vi "Set Injected Value.vi"(8 "error in (no error)":errorcluster, 10 "Value":T1, 11 "Fault-Injection_Boolean in":refnum<class "Fault-Injection_U64.lvclass">) -> (0 "error out":errorcluster, 3 "Fault-Injection_Boolean out":refnum<class "Fault-Injection_U64.lvclass">)   [LabVIEW 2021, in "Fault-Injection_U64.lvclass"]
uses:
  Fault-Injection_U64.lvclass
  Support/Value Type.ctl
  Fault-Injection_U64.lvclass/Fault-Injection_U64.ctl
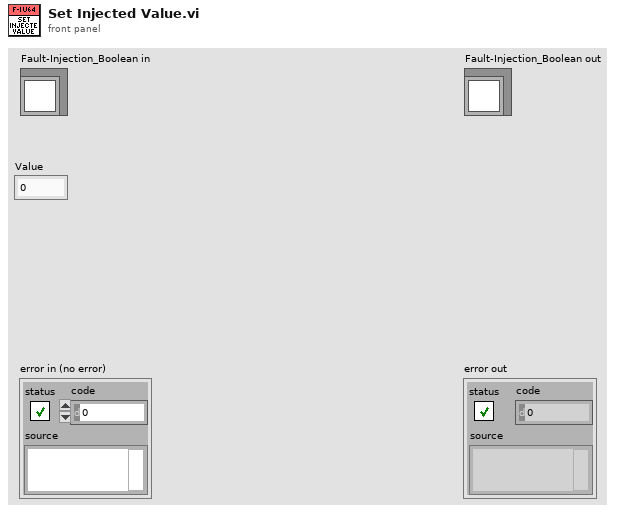
[diagram p1: front panel]
types:
  T1 = typedef "Fault-Injection_U64.lvclass/Value Type.ctl" = u64
  T2 = typedef "Fault-Injection_U64.lvclass/DVR Type.ctl" = cluster{"Enable":bool, "Injected Value":T1, "Value":T3}
  T3 = typedef "Fault-Injection_U64.lvclass/Abs Class Type.ctl" = refnum<class "Abs_U64 Integer.lvclass">
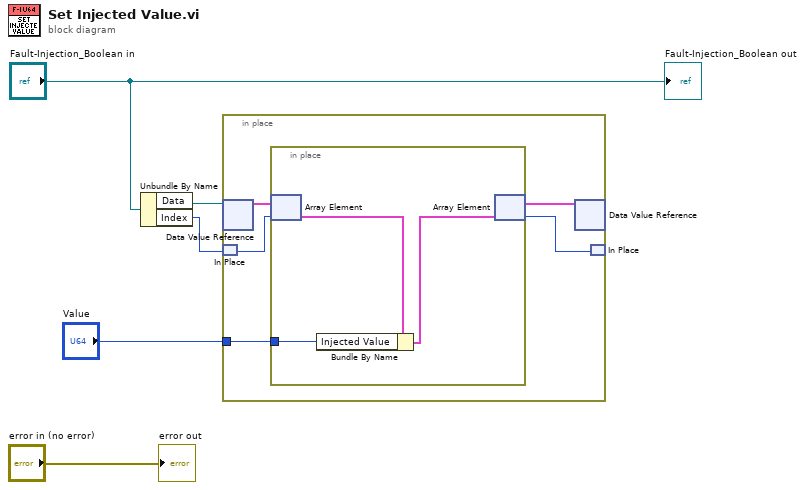
[diagram p0: block diagram]
diagram:
  n1 = Unbundle By Name("Fault-Injection_Boolean in") -> ("Data"=w4:refnum<data-value>, "Index"=w3:i32)
  n2 = in-place {
    in-place-border: "Value" -> [w6]
    n3 = in-place-dvr #1(w4) -> (w10:T2[])  [unwired: 1 out]
    n4 = in-place-match #2(w3) -> (w8:i32)
    n5 = in-place {
      in-place-border: w6 -> [w11]
      n6 = in-place-array #3(w10, w8) -> (w13:T2)
      n7 = Bundle By Name(cluster=w13, "Injected Value"=w11) -> (w12:T2)
      n8 = in-place-array #3(w12) -> (w9:T2[], w7:i32)
    }
    n9 = in-place-dvr #1(w9) -> ()  [unwired: 2 out]
    n10 = in-place-match #2(w7) -> ()  [unwired: 1 out]
  }
  "error out" <- "error in (no error)"
  "Fault-Injection_Boolean out" <- "Fault-Injection_Boolean in"
